vi "Create CAN Outgoing Section.vi"(8 "error in (no error)":errorcluster, 11 "Parent Ref in":T1 format="%.0x") -> (0 "error out":errorcluster, 3 "Parent Ref out":T1 format="%.0x")   [LabVIEW 2015, in "J1939 Addon Shared.lvlib"]
uses:
  J1939 Addon Shared.lvlib
  <vilib>/NI Veristand/Custom Device API/Custom Device Item Ref.ctl
  Constants.vi
  <vilib>/NI/NIVS System Definition Utilities/System Definition Utilities.lvlib
  <vilib>/NI VeriStand/Custom Device API/Custom Device API.lvlib
panel:
  # "OUTPUTS"
  # "INPUTS"
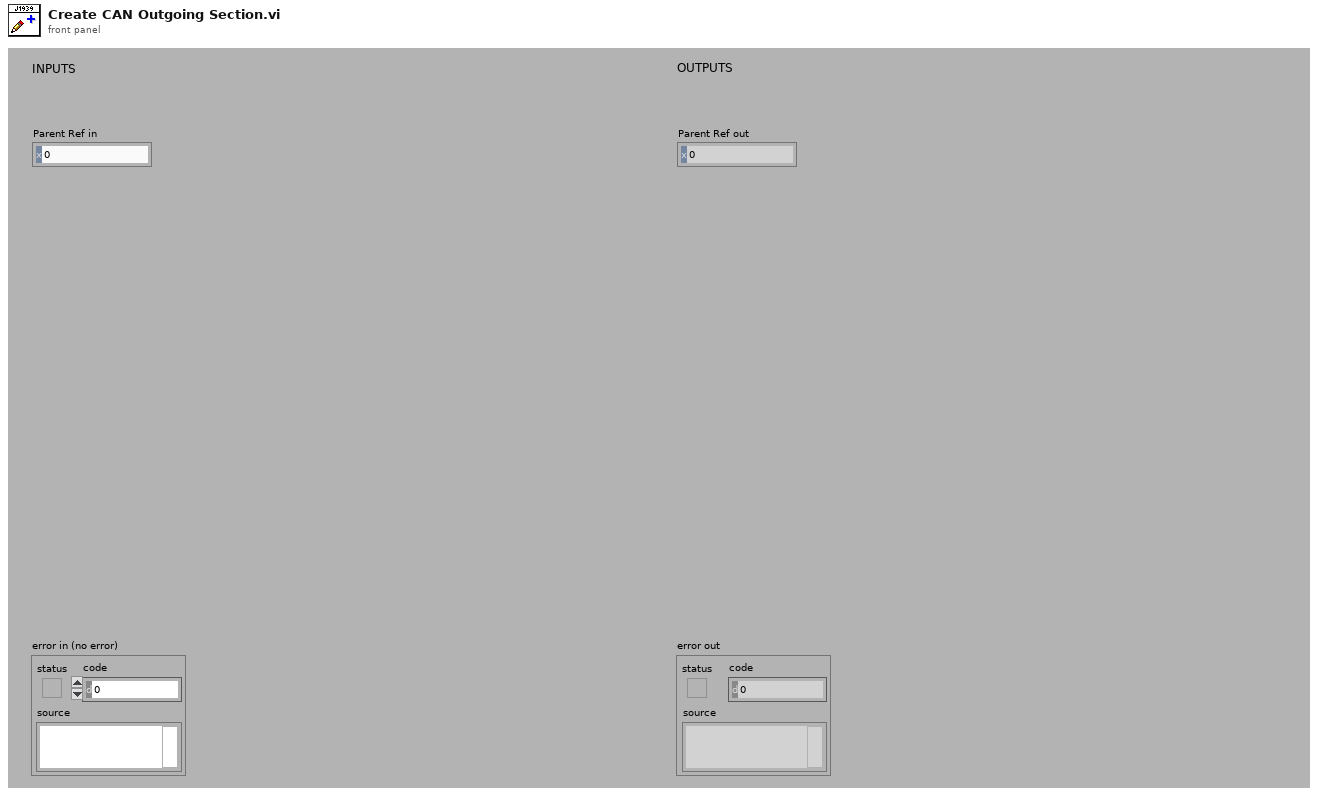
[diagram p1: front panel]
types:
  T1 = typedef "Custom Device API.lvlib/Custom Device Item Ref.ctl" = u64
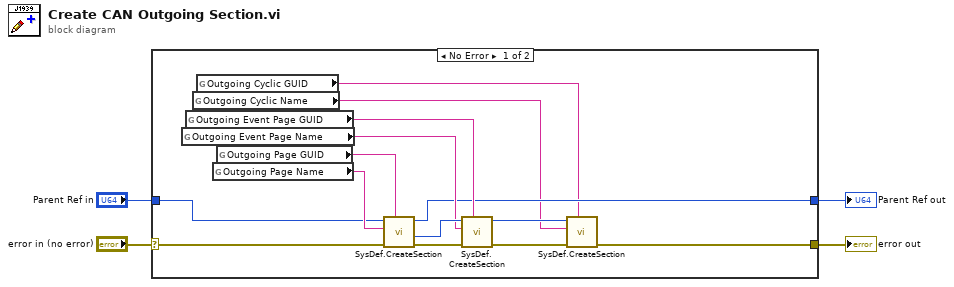
[diagram p0: block diagram]
diagram:
  n1 = case shown="No Error" "error in (no error)" {
    selector: "error in (no error)" -> [w12 w20]
    tunnel: [w8 w20] -> w3
    tunnel: "Parent Ref in" -> [w11 w19]
    tunnel: [w10 w19] -> w1
    frame No Error {
      n2 = global read "Constants.vi" "Outgoing Event Page Name"() -> (w13:string)
      n3 = global read "Constants.vi" "Outgoing Event Page GUID"() -> (w14:string)
      n4 = global read "Constants.vi" "Outgoing Cyclic Name"() -> (w5:string)
      n5 = global read "Constants.vi" "Outgoing Cyclic GUID"() -> (w6:string)
      n6 = global read "Constants.vi" "Outgoing Page Name"() -> (w15:string)
      n7 = global read "Constants.vi" "Outgoing Page GUID"() -> (w16:string)
      n8 = call <vilib>:"SysDef.CreateSection.vi"("GUID"=w16, "error in (no error)"=w12, "Name"=w15, "nodeID"=w11) -> ("error out"=w18:errorcluster, "New NodeID"=w17:u64, "nodeID out"=w10:u64)  [unwired: 4 in, 1 out]
      n9 = call <vilib>:"SysDef.CreateSection.vi"("GUID"=w14, "error in (no error)"=w18, "Name"=w13, "nodeID"=w17) -> ("error out"=w9:errorcluster, "nodeID out"=w7:u64)  [unwired: 4 in, 2 out]
      n10 = call <vilib>:"SysDef.CreateSection.vi"("GUID"=w6, "error in (no error)"=w9, "Name"=w5, "nodeID"=w7) -> ("error out"=w8:errorcluster)  [unwired: 4 in, 3 out]
    }
    frame Error {
    }
  }
  "error out" <- w3
  "Parent Ref out" <- w1
